vi "3-3.vi"() -> ()   [LabVIEW 2017]
panel:
  out "输出3":dbl
  in  "偏移量3":dbl
  in  "长度2":dbl
  in  "偏移量2":dbl
  in  "长度":dbl
  in  "偏移量":dbl
  out "输出2":string
  out "输出 1":string
  in  "输入":string
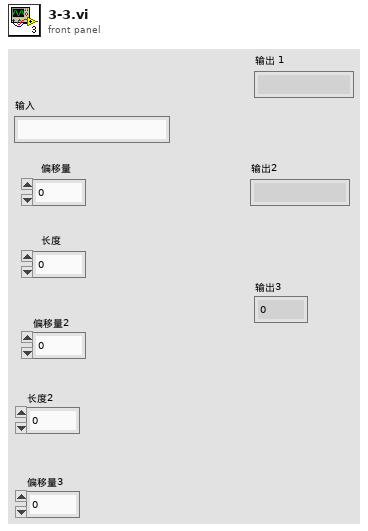
[diagram p1: front panel]
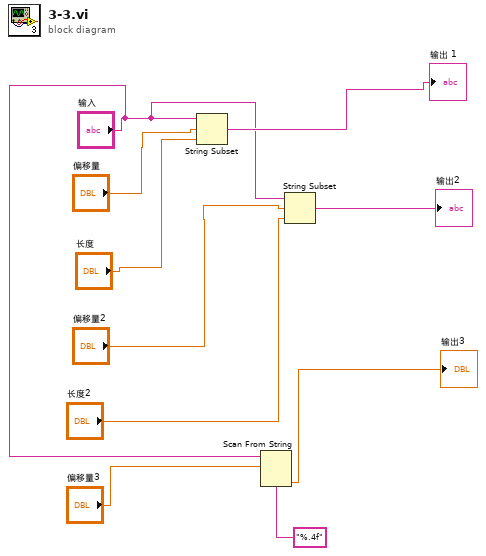
[diagram p0: block diagram]
diagram:
  n1 = String Subset(string="输入", offset (0)="偏移量", length (rest)="长度") -> (substring=→"输出 1":string)
  n2 = Scan From String(format string="%.4f" ("格式字符串"), input string="输入", initial scan location="偏移量3") -> (output 1=→"输出3":dbl)  [unwired: 2 in, 3 out]
  n3 = String Subset(string="输入", offset (0)="偏移量2", length (rest)="长度2") -> (substring=→"输出2":string)
